vi "GetTACWindowIngoHeucke.vi"(0 "Enum":enum16{"ini", "get", "quick"}(ring), 4 "auto":bool) -> (1 "TAC.Window (diff)":u16, 2 "Waveform Graph 2":refnum<vi>, 3 "Decays":u32[][](graph), 5 "TAC.Window (min)":u16, 6 "allchan?":bool, 7 "Cursor.Cursor Position:Cursor X":u16, 8 "Cursor.Cursor Position:Cursor X 2":u16, 9 "x-values":dbl[](array[numeric]) format="%.2f", 10 "ready?":bool)   [LabVIEW 2009]
uses:
  IMAGE Cluster 2.ctl
panel:
  out "TAC.TAC Range (ns)":sgl
  out "# microchannels":i32
  in  "ADC-Resolution":u16(ring) items=["8bit", "12bit", "4bit", "15bit"]
  in  "Ring":u8(ring) items=["linear y-axis", "log y-axis"]
  out "Boolean 2":bool
  out "TAC-Cube (for Spotfinder)":T1(ring)=enum."no Spotfinding"
  in  "OK Button":bool
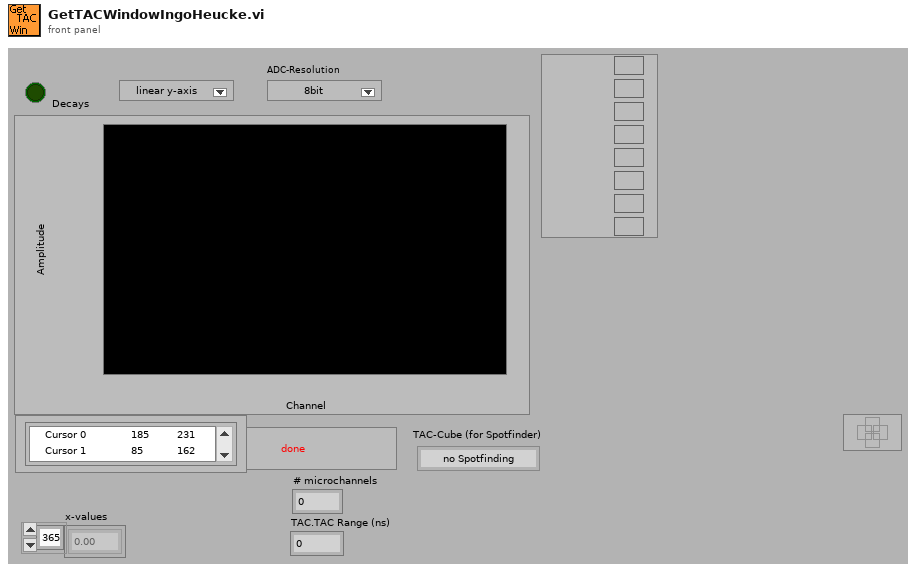
[diagram p1: front panel]
types:
  T1 = enum16{"1", "2", "3", "4", "5", "6", "7", "Sum", "no Spotfinding", "Separation"}
  T2 = typedef "IMAGE Cluster 2.ctl" = cluster{"decay":u16[][][][][], "sum of photons":u32[][][][]}
  T3 = typedef "FIFOSettings_BH.ctt" = cluster{"Measurement":cluster{"Binning (ms)":sgl, "External Trigger Condition":u16, "Stop Condition:":u16, "Stop Count":dbl, "Buffer Size (Photons)":u16, "No of Channels":u16, "Ext Latch Delay":i16}, "ADC":cluster{"Module":u16, "ADC Resolution":i32, "Dither Range":i16, "Count Increment":i16, "Macro Time Clock":i16}, "SYNC":cluster{"SYNC ZC Level (mV)":sgl, "SYNC Freq Divider":i16, "SYNC Holdoff (ns)":sgl, "SYNC Threshold (mV)":sgl}, "TAC":cluster{"TAC Range (ns)":sgl, "TAC Gain":i16, "TAC Offset (%)":sgl, "TAC Limit Low (%)":sgl, "TAC Limit High (%)":sgl}, "CFD":cluster{"CFD Limit Low (mV)":sgl, "CFD Limit High (mV)":sgl, "CFD ZC Level (mV)":sgl, "CFD Holdoff (ns)":sgl}}
  T4 = typedef "Settings.ctl" = cluster{"threshold":cluster{"max":u32, "min":u32}, "RGB or false color":bool, "16bit":bool, "log/lin axis":u16, "spotsize button":bool, "Pixelsize":u16, "autoscale x":bool, "autoscale y":bool, "correlation":bool, "ADC-Resolution":i32, "F2-lifetime":cluster{"display tau":bool, "display F2":bool, "Palette Number lifetime":enum32{"Gray", "Binary", "Gradient", "Rainbow", "Temperature"}, "Palette Number F2":enum32{"Gray", "Binary", "Gradient", "Rainbow", "Temperature"}, "max tau-Value":dbl, "min tau-Value":dbl, "max F2-Value":dbl, "min F2-Value":dbl}, "TAC-Window 1":u16, "TAC-Window 2":u16, "false color palette":cluster{"1":u32, "2":u32, "3":u32, "4":u32, "5":u32, "6":u32, "7":u32, "8":u32, "8 2":u32, "8 3":u32, "8 4":u32, "8 5":u32}}
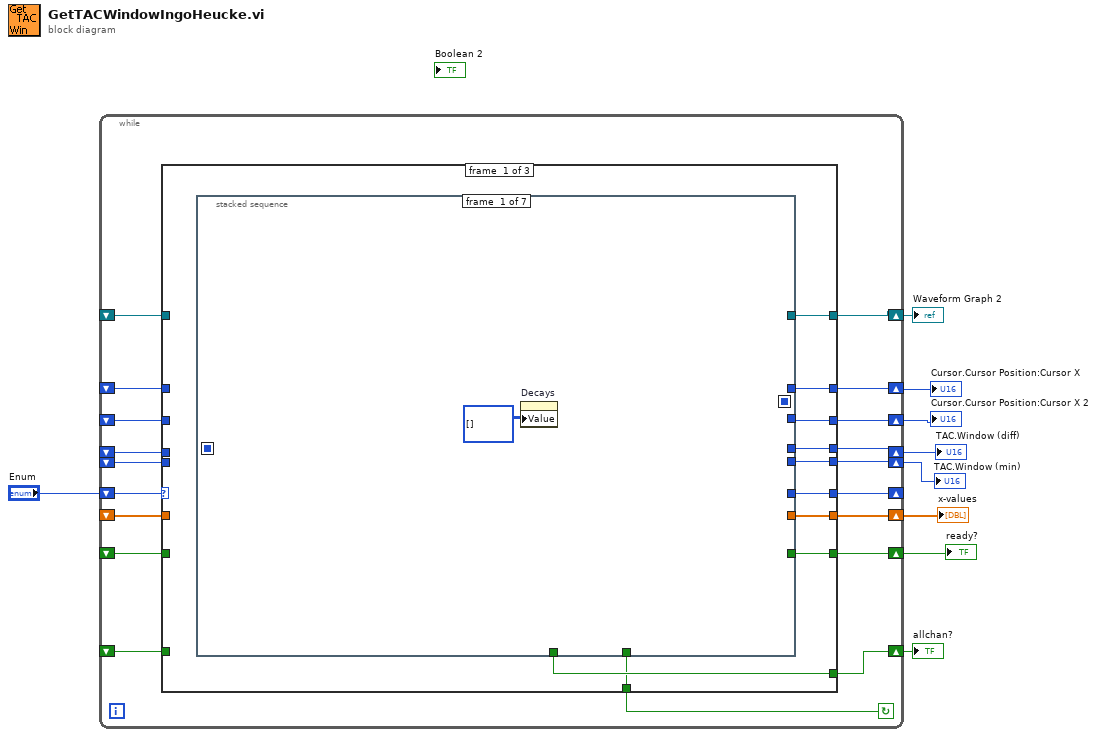
[diagram p0: block diagram]
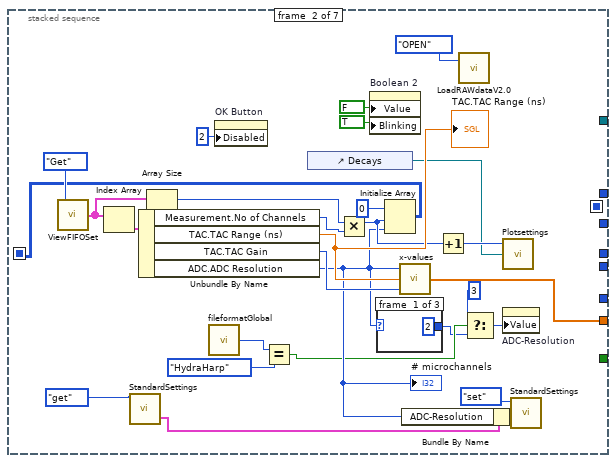
[diagram p2: hidden frame]
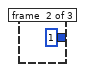
[diagram p3: hidden frame]
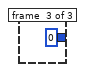
[diagram p4: hidden frame]
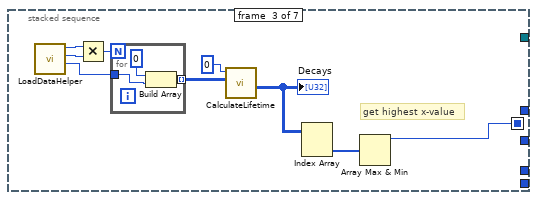
[diagram p5: hidden frame]
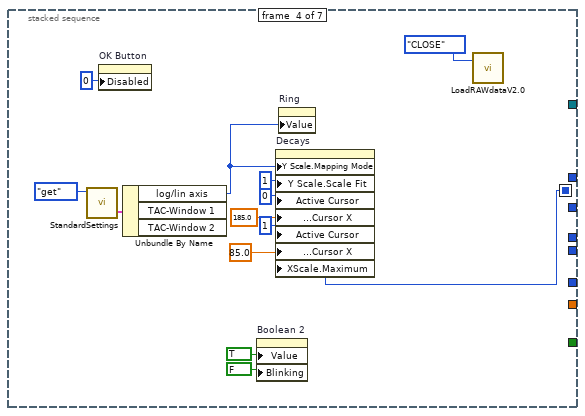
[diagram p6: hidden frame]
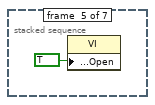
[diagram p7: hidden frame]
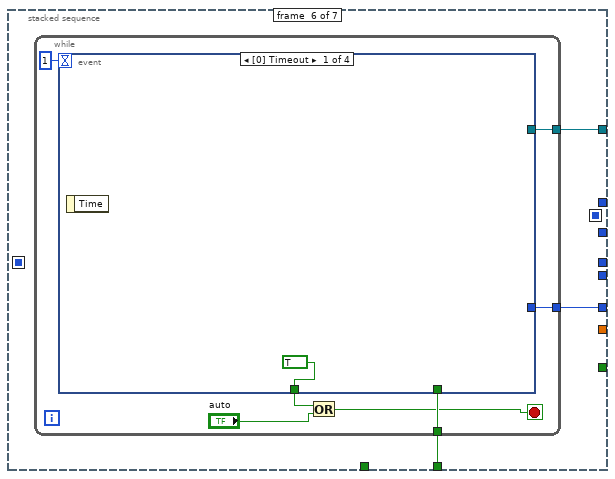
[diagram p8: hidden frame]
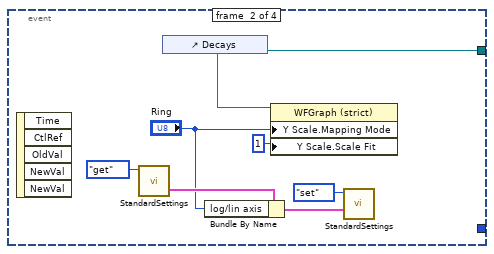
[diagram p9: hidden frame]
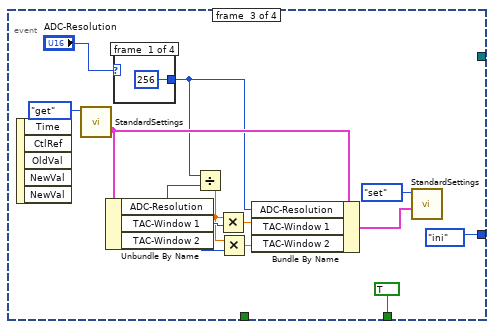
[diagram p10: hidden frame]
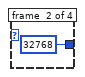
[diagram p11: hidden frame]
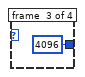
[diagram p12: hidden frame]
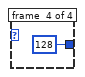
[diagram p13: hidden frame]
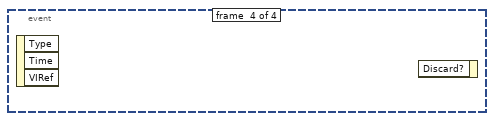
[diagram p14: hidden frame]
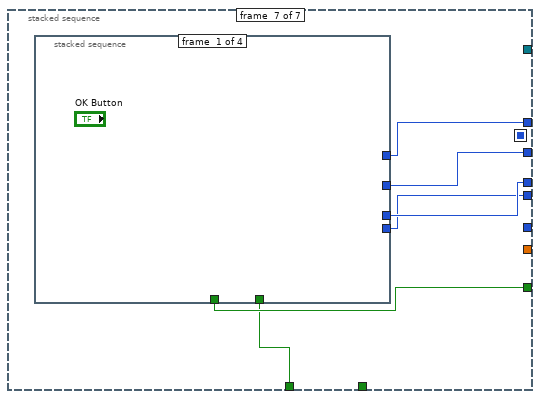
[diagram p15: hidden frame]
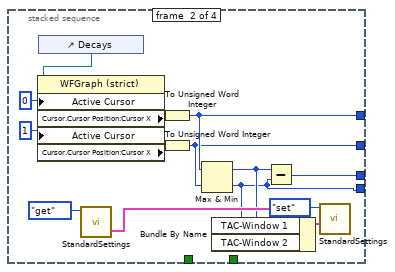
[diagram p16: hidden frame]
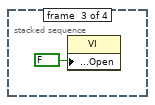
[diagram p17: hidden frame]
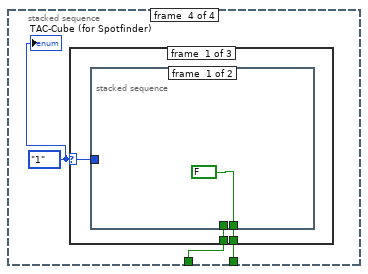
[diagram p18: hidden frame]
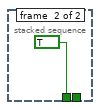
[diagram p19: hidden frame]
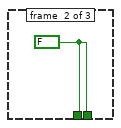
[diagram p20: hidden frame]
diagram:
  n1 = while {
    shift-right: [w28] -> w8
    shift-left: _ -> [w26]
    shift-right: [w27] -> w9
    shift-left: _ -> [w25]
    shift-right: [w24] -> w7
    shift-left: _ -> [w23]
    shift-right: [w21] -> w5
    shift-left: _ -> [w19]
    shift-right: [w22] -> w6
    shift-left: _ -> [w20]
    shift-right: [w13] -> w4
    shift-left: _ -> [w18]
    shift-right: [w17] -> w3
    shift-left: _ -> [w16]
    shift-right: [w15] -> w2
    shift-left: _ -> [w14]
    shift-right: [w10] -> _
    shift-left: "Enum" -> [w11]
    stop <- w12 continue-if-true
    n2 = case shown="\"ini\", Default" w11 {
      tunnel: [w38 w175 w189] -> w28
      tunnel: [w37 w174 w188] -> w27
      tunnel: w26 -> [_ w175 _]
      tunnel: w25 -> [_ w174 _]
      tunnel: [w36 w173 w177] -> w24
      tunnel: w23 -> [_ w173 _]
      tunnel: [w35 w172 w194] -> w22
      tunnel: [w34 w171 w195] -> w21
      tunnel: w20 -> [_ w172 w194]
      tunnel: w19 -> [_ w171 w195]
      tunnel: [w33 w170 w196] -> w13
      tunnel: w18 -> [_ w170 w196]
      tunnel: [w32 w169 w193] -> w17
      tunnel: w16 -> [_ w169 w193]
      tunnel: [w31 w168 w192] -> w15
      tunnel: w14 -> [_ w168 w192]
      tunnel: [w30 _ _] -> w12
      tunnel: [w29 _ _] -> w10
      frame #0 {
        n3 = stacked-sequence {
          seq-local: [_ w65 _ _ _ _ _] -> [_ _ _ _ _ _ _]
          seq-local: [_ _ w71 _ _ _ _] -> [_ _ _ w84 _ _ _]
          tunnel: [_ _ _ _ _ _ w138] -> w38
          tunnel: [_ _ _ _ _ _ w137] -> w37
          tunnel: [_ w40 _ _ _ _ _] -> w36
          tunnel: [_ _ _ _ _ _ w136] -> w35
          tunnel: [_ _ _ _ _ _ w135] -> w34
          tunnel: [_ _ _ _ _ _ w134] -> w33
          tunnel: [_ _ _ _ _ w99 _] -> w32
          tunnel: [_ _ _ _ _ _ w133] -> w31
          tunnel: [_ _ _ _ _ w98 _] -> w30
          tunnel: [_ _ _ _ _ w97 _] -> w29
          frame #0 {
            n4 = property on="Decays" class="WFGraph (strict)"("Value"=u32[][] [] ("Waveform Graph")) -> ()  [unwired: 2 in, 2 out]
          }
          frame #1 {
            n5 = call "ViewFIFOSet.vi"("Enum"=enum16{"Display", "change", "Get", "Set"}."Get") -> ("FIFO Settings (Array)"=w51:T3[])  [unwired: 1 in]
            n6 = Index Array(array=w51) -> (element=w52:T3)  [unwired: 1 in]
            n7 = call "StandardSettings.vi"("Enum"=enum16{"Load", "get", "Save", "set"}."get") -> ("StandardSettings"=w57:T4)  [unwired: 4 in]
            n8 = Unbundle By Name(w52) -> ("Measurement.No of Channels"=w50:u16, "TAC.TAC Range (ns)"=w61:sgl, "TAC.TAC Gain"=w60:i16, "ADC.ADC Resolution"=w47:i32)
            "# microchannels" <- w47
            "TAC.TAC Range (ns)" <- w61
            n9 = Array Size(array=w51) -> (size(s)=w49:i32)
            n10 = call "fileformatGlobal.vi"() -> ("fileformat out"=w46:enum16{"Herty", "Ken", "SPC130", "HydraHarp"})  [unwired: 2 in]
            n11 = property on="OK Button" class="Boolean"("Disabled"=u8 2) -> ()  [unwired: 2 in, 2 out]
            n12 = Equal?(x=w46, y=enum16{"Herty", "Ken", "SPC130", "HydraHarp"}."HydraHarp") -> (x = y?=w43:bool)
            n13 = control-ref of="Decays"() -> (w53:refnum<vi>)
            n14 = Multiply(x=w49, y=w50) -> (x*y=w48:i32)
            n15 = property on="Boolean 2" class="Boolean (strict)"("Value"=FALSE ("Boolean 2"), "Blinking"=TRUE) -> ()  [unwired: 2 in, 2 out]
            n16 = case shown="128, Default" w47 {
              tunnel: [u16 2 u16 1 u16 0] -> w42
              frame #0 {
              }
              frame #1 {
              }
              frame #2 {
              }
            }
            n17 = Initialize Array(u32 0 ("element"), w48, w47) -> (w65:u32[][])
            n18 = call "x-values.vi"("TAC Gain"=w60, "TAC Rang [ns]"=w61, "No. Microchannel"=w47) -> ("Array"=w40:dbl[])
            n19 = Bundle By Name(cluster=w57, "ADC-Resolution"=w47) -> (w58:T4)
            n20 = Increment(x=w48) -> (x+1=w55:i32)
            n21 = call "LoadRAWdataV2.0.vi"("action"=enum16{"OPEN", "READ", "CLOSE"}."OPEN" ("Enum")) -> ()  [unwired: 1 in, 2 out]
            n22 = Select(t=u16 3, s=w43, f=w42) -> (s? t:f=w44:u16)
            n23 = call "Plotsettings.vi"("Decays 2"=w53, "No of Channels"=w55) -> ()  [unwired: 4 in]
            n24 = property on="ADC-Resolution" class="Ring (strict)"("Value"=w44) -> ()  [unwired: 2 in, 2 out]
            n25 = call "StandardSettings.vi"("StandardSettings"=w58, "Enum"=enum16{"Load", "get", "Save", "set"}."set") -> ()  [unwired: 3 in, 1 out]
          }
          frame #2 {
            # "get highest x-value"
            n26 = call "LoadDataHelper.vi"() -> ("pixel per line"=w75:u32, "planes"=w76:u32, "lines"=w77:u32)  [unwired: 7 in, 2 out]
            n27 = Multiply(x=w77, y=w76) -> (x*y=w78:u32)
            n28 = for {
              N: w78 -> [_]
              tunnel: w75 -> [w81]
              tunnel: [w80] -> w74 mode=indexing
              n29 = Build Array(0 ("starting y-point"), w81) -> (w80:u32[])
            }
            n30 = call "CalculateLifetime.vi"("Pos Array"=w74, "starting y-point"=0) -> ("Decay"=w73:u32[][])  [unwired: 5 in]
            "Decays" <- w73
            n31 = Index Array(array=w73) -> (element=w72:u32[])  [unwired: 2 in]
            n32 = Array Max & Min(array=w72) -> (max value=w71:u32)  [unwired: 3 out]
          }
          frame #3 {
            n33 = call "StandardSettings.vi"("Enum"=enum16{"Load", "get", "Save", "set"}."get") -> ("StandardSettings"=w90:T4)  [unwired: 4 in]
            n34 = property on="OK Button" class="Boolean"("Disabled"=u8 0) -> ()  [unwired: 2 in, 2 out]
            n35 = Unbundle By Name(w90) -> ("log/lin axis"=w86:u16)  [unwired: 2 out]
            n36 = property on="Boolean 2" class="Boolean (strict)"("Value"=TRUE ("Boolean 2"), "Blinking"=FALSE) -> ()  [unwired: 2 in, 2 out]
            n37 = property on="Decays" class="WFGraph (strict)"("Y Scale.Mapping Mode"=w86, "Y Scale.Scale Fit"=u8 1, "Active Cursor"=u32 0, "Cursor.Cursor Position:Cursor X"=185.0, "Active Cursor"=u32 1, "Cursor.Cursor Position:Cursor X"=85.0, "XScale.Maximum"=w84) -> ()  [unwired: 2 in, 2 out]
            n38 = property on="Ring" class="Ring (strict)"("Value"=w86) -> ()  [unwired: 2 in, 2 out]
            n39 = call "LoadRAWdataV2.0.vi"("action"=enum16{"OPEN", "READ", "CLOSE"}."CLOSE" ("Enum")) -> ()  [unwired: 1 in, 2 out]
          }
          frame #4 {
            n40 = property class="VI"("Front Panel Window:Open"=TRUE) -> ()  [unwired: 2 in, 2 out]
          }
          frame #5 {
            n41 = while {
              tunnel: [w106] -> w99
              tunnel: [w105] -> w98
              tunnel: [w104] -> w97
              stop <- w102 stop-if-true
              n42 = event shown="[0] Timeout" {
                selector: _ -> [_ _ _ _]
                dyn-events: _ -> [_ _ _ _]
                timeout: 1 -> [_ _ _ _]
                tunnel: [_ w114 _ _] -> w106
                tunnel: [_ _ TRUE _] -> w105
                tunnel: [_ _ enum16{"ini", "get", "quick"}."ini" ("Enum") _] -> w104
                tunnel: [TRUE _ _ _] -> w101
                event #0 {
                  n43 = event-data() -> ()  [unwired: 1 in, 1 out]
                }
                event #1 {
                  n44 = event-data() -> ()  [unwired: 1 in, 5 out]
                  n45 = call "StandardSettings.vi"("Enum"=enum16{"Load", "get", "Save", "set"}."get") -> ("StandardSettings"=w111:T4)  [unwired: 4 in]
                  n46 = control-ref of="Decays"() -> (w114:refnum<vi>)
                  n47 = Bundle By Name(cluster=w111, "log/lin axis"="Ring") -> (w110:T4)
                  n48 = property class="WFGraph (strict)"(reference=w114, "Y Scale.Mapping Mode"="Ring", "Y Scale.Scale Fit"=u8 1) -> ()  [unwired: 1 in, 2 out]
                  n49 = call "StandardSettings.vi"("StandardSettings"=w110, "Enum"=enum16{"Load", "get", "Save", "set"}."set") -> ()  [unwired: 3 in, 1 out]
                }
                event #2 {
                  n50 = event-data() -> ()  [unwired: 1 in, 5 out]
                  n51 = call "StandardSettings.vi"("Enum"=enum16{"Load", "get", "Save", "set"}."get") -> ("StandardSettings"=w125:T4)  [unwired: 4 in]
                  n52 = Unbundle By Name(w125) -> ("ADC-Resolution"=w115:i32, "TAC-Window 1"=w120:u16, "TAC-Window 2"=w121:u16)
                  n53 = case shown="3" "ADC-Resolution" {
                    tunnel: [256 32768 4096 128] -> w116
                    frame #0 {
                    }
                    frame #1 {
                    }
                    frame #2 {
                    }
                    frame #3 {
                    }
                  }
                  n54 = Divide(x=w116, y=w115) -> (x/y=w119:dbl)
                  n55 = Multiply(x=w119, y=w120) -> (x*y=w118:dbl)
                  n56 = Multiply(x=w119, y=w121) -> (x*y=w117:dbl)
                  n57 = Bundle By Name(cluster=w125, "ADC-Resolution"=w116, "TAC-Window 1"=w118, "TAC-Window 2"=w117) -> (w124:T4)
                  n58 = call "StandardSettings.vi"("StandardSettings"=w124, "Enum"=enum16{"Load", "get", "Save", "set"}."set") -> ()  [unwired: 3 in, 1 out]
                }
                event #3 {
                  n59 = event-data() -> ()  [unwired: 1 in, 3 out]
                  n60 = event-data() -> ()  [unwired: 2 in, 1 out]
                }
              }
              n61 = Or(x=w101, y="auto") -> (x .or. y?=w102:bool)
            }
          }
          frame #6 {
            n62 = stacked-sequence {
              tunnel: [_ w142 _ _] -> w138
              tunnel: [_ w141 _ _] -> w137
              tunnel: [_ w148 _ _] -> w136
              tunnel: [_ w139 _ _] -> w135
              tunnel: [_ _ _ w156] -> w134
              tunnel: [_ _ _ w155] -> w133
              frame #0 {
              }
              frame #1 {
                n63 = control-ref of="Decays"() -> (w147:refnum<vi>)
                n64 = property class="WFGraph (strict)"(reference=w147, "Active Cursor"=u32 0, "Active Cursor"=u32 1) -> ("Cursor.Cursor Position:Cursor X"=w150:dbl, "Cursor.Cursor Position:Cursor X"=w149:dbl)  [unwired: 1 in, 2 out]
                n65 = call "StandardSettings.vi"("Enum"=enum16{"Load", "get", "Save", "set"}."get") -> ("StandardSettings"=w144:T4)  [unwired: 4 in]
                n66 = To Unsigned Word Integer(number=w150) -> (unsigned 16bit integer=w142:u16)
                n67 = To Unsigned Word Integer(number=w149) -> (unsigned 16bit integer=w141:u16)
                n68 = Max & Min(x=w142, y=w141) -> (max(x,y)=w140:u16, min(x,y)=w139:u16)
                n69 = Bundle By Name(cluster=w144, "TAC-Window 1"=w140, "TAC-Window 2"=w139) -> (w143:T4)
                n70 = Subtract(x=w140, y=w139) -> (x-y=w148:u16)
                n71 = call "StandardSettings.vi"("StandardSettings"=w143, "Enum"=enum16{"Load", "get", "Save", "set"}."set") -> ()  [unwired: 3 in, 1 out]
              }
              frame #2 {
                n72 = property class="VI"("Front Panel Window:Open"=FALSE) -> ()  [unwired: 2 in, 2 out]
              }
              frame #3 {
                w154 = T1."1" ("TAC-Cube (for Spotfinder)")
                n73 = case shown="\"1\", Default" w154 {
                  selector: w154 -> [w159 _ _]
                  tunnel: [w158 w162 w164] -> w156
                  tunnel: [w157 w162 w163] -> w155
                  frame #0 {
                    n74 = stacked-sequence {
                      tunnel: w159 -> [_ _]
                      tunnel: [_ TRUE] -> w158
                      tunnel: [FALSE ("allchan?") _] -> w157
                      frame #0 {
                      }
                      frame #1 {
                      }
                    }
                  }
                  frame #1 {
                    w162 = FALSE
                  }
                  frame #2 {
                    n75 = stacked-sequence {
                      tunnel: [w165 _] -> w164
                      tunnel: [w165 _] -> w163
                      frame #0 {
                        w165 = TRUE ("allchan?")
                      }
                      frame #1 {
                        n76 = call "IMAGECluster.vi"("set?"=TRUE, "IMAGE Cluster in"=T2 {"decay"=[], "sum of photons"=[]} ("IMAGE Cluster (input)")) -> ()  [unwired: 1 out]
                      }
                    }
                  }
                }
                "TAC-Cube (for Spotfinder)" <- w154
              }
            }
          }
        }
      }
      frame #1 {
      }
      frame #2 {
        n77 = call "ViewFIFOSet.vi"("Enum"=enum16{"Display", "change", "Get", "Set"}."Get") -> ("FIFO Settings (Array)"=w197:T3[])  [unwired: 1 in]
        n78 = call "StandardSettings.vi"("Enum"=enum16{"Load", "get", "Save", "set"}."get") -> ("StandardSettings"=w190:T4)  [unwired: 4 in]
        n79 = Index Array(array=w197) -> (element=w176:T3)  [unwired: 1 in]
        n80 = Unbundle By Name(w190) -> ("TAC-Window 1"=w189:u16, "TAC-Window 2"=w188:u16, "ADC-Resolution"=w180:i32)
        n81 = Unbundle By Name(w176) -> ("ADC.ADC Resolution"=w179:i32, "TAC.TAC Range (ns)"=w181:sgl, "TAC.TAC Gain"=w182:i16)
        n82 = Not Equal To 0?(x=w179) -> (x != 0?=w186:bool)
        n83 = Select(t=4096, s=w186, f=256) -> (s? t:f=w178:i32)
        n84 = Greater?(x=w178, y=w180) -> (0:w184:bool)
        n85 = Select(t=w180, s=w184, f=w178) -> (s? t:f=w183:i32)
        n86 = call "x-values.vi"("TAC Gain"=w182, "TAC Rang [ns]"=w181, "No. Microchannel"=w183) -> ("Array"=w177:dbl[])
      }
    }
  }
  "Cursor.Cursor Position:Cursor X 2" <- w9
  "Cursor.Cursor Position:Cursor X" <- w8
  "x-values" <- w7
  "TAC.Window (diff)" <- w6
  "TAC.Window (min)" <- w5
  "ready?" <- w4
  "Waveform Graph 2" <- w3
  "allchan?" <- w2
